vi "Convert - NaN String.vi"(10 "Replacement":string="-", 11 "Strings in":string[](array[string])) -> (3 "Converted Strings":string[](array[string]))   [LabVIEW 2015, in "Utility.lvlib"]
uses:
  Utility.lvlib
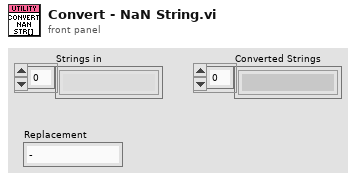
[diagram p1: front panel]
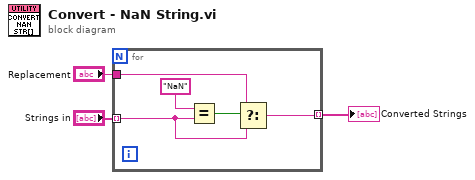
[diagram p0: block diagram]
diagram:
  n1 = for {
    tunnel: "Strings in" -> [w7] mode=indexing
    tunnel: [w6] -> w3 mode=indexing
    tunnel: "Replacement" -> [w4]
    n2 = Equal?(x="NaN", y=w7) -> (x = y?=w8:bool)
    n3 = Select(t=w4, s=w8, f=w7) -> (s? t:f=w6:string)
  }
  "Converted Strings" <- w3
